vi "Overlay Circles.vi"(7 "Group":string, 8 "error in":errorcluster, 9 "Einstellungen":T1={"Farbe Kreis"=6618880, "Kreis ausfüllen?"=FALSE, "Bounding Rechteck anzeigen?"=FALSE, "Farbe Bounding Rechteck"=16711680}, 10 "Circles":T3(array[cluster]), 11 "Image in":T2) -> (0 "error out":errorcluster, 3 "Image out":T2)   [LabVIEW 2024]
uses:
  Kontaktmontagemodul.exe/1abvi3w/vi.lib/vision/Image Controls.llb/IMAQ Image.ctl
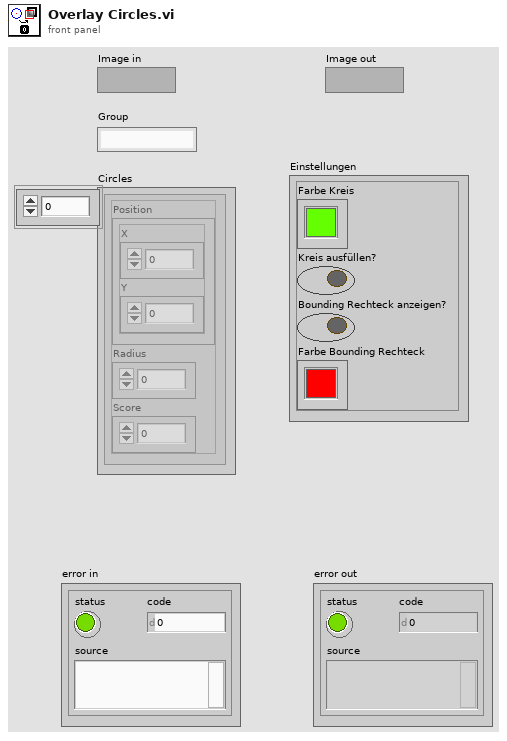
[diagram p1: front panel]
types:
  T1 = cluster{"Farbe Kreis":u32, "Kreis ausfüllen?":bool, "Bounding Rechteck anzeigen?":bool, "Farbe Bounding Rechteck":u32}
  T2 = typedef "IMAQ Image.ctl" = refnum<image>
  T3 = cluster{"Position":cluster{"X":sgl, "Y":sgl}, "Radius":dbl, "Score":dbl}[]
  T4 = cluster{"Left":i32, "Top":i32, "Right":i32, "Bottom":i32}
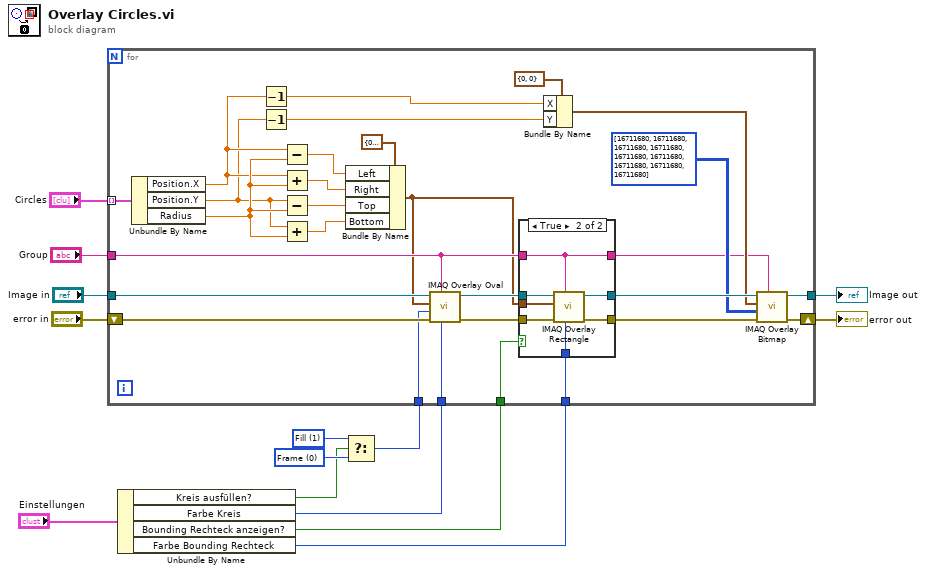
[diagram p0: block diagram]
diagram:
  w7 = u32 1 items=["Frame", "Fill"] ("Drawing Mode (Frame)")
  w8 = u32 0 items=["Frame", "Fill"] ("Drawing Mode (Frame)")
  n1 = Unbundle By Name("Einstellungen") -> ("Kreis ausfüllen?"=w5:bool, "Farbe Kreis"=w4:u32, "Bounding Rechteck anzeigen?"=w3:bool, "Farbe Bounding Rechteck"=w2:u32)
  n2 = Select(t=w7, s=w5, f=w8) -> (s? t:f=w6:u32)
  n3 = for {
    tunnel: "Circles" -> [w43] mode=indexing
    shift-right: [w15] -> w10
    shift-left: "error in" -> [w35]
    tunnel: "Image in" -> [w36]
    tunnel: [w17] -> w12
    tunnel: w4 -> [w23]
    tunnel: w6 -> [w22]
    tunnel: w3 -> [w21]
    tunnel: w2 -> [w20]
    tunnel: "Group" -> [w19]
    n4 = Unbundle By Name(w43) -> ("Position.X"=w28:sgl, "Position.Y"=w27:sgl, "Radius"=w41:dbl)
    n5 = Decrement(x=w28) -> (x-1=w26:sgl)
    n6 = Decrement(x=w27) -> (x-1=w25:sgl)
    n7 = Subtract(x=w28, y=w41) -> (x-y=w37:dbl)
    n8 = Add(x=w28, y=w41) -> (x+y=w38:dbl)
    n9 = Subtract(x=w27, y=w41) -> (x-y=w40:dbl)
    n10 = Add(x=w27, y=w41) -> (x+y=w39:dbl)
    n11 = Bundle By Name(cluster=T4 {"Left"=0, "Top"=0, "Right"=0, "Bottom"=0} ("Rectangle"), "Left"=w37, "Right"=w38, "Top"=w40, "Bottom"=w39) -> (w16:T4)
    n12 = call "IMAQ Overlay Oval"("Color"=w23, "Group"=w19, "error in (no error)"=w35, "Drawing Mode (Frame)"=w22, "Bounding Rectangle"=w16, "Image"=w36) -> ("error out"=w33:errorcluster, "Image Out"=w34:T2)  [unwired: 4 in]
    n13 = case shown="True" w21 {
      tunnel: w34 -> [w46 w53]
      tunnel: w33 -> [w45 w52]
      tunnel: w16 -> [_ w51]
      tunnel: [w46 w50] -> w32
      tunnel: [w45 w49] -> w31
      tunnel: w20 -> [_ w48]
      tunnel: w19 -> [w44 w47]
      tunnel: [w44 w47] -> w18
      frame False {
      }
      frame True {
        n14 = call "IMAQ Overlay Rectangle"("Color"=w48, "Group"=w47, "error in (no error)"=w52, "Rectangle"=w51, "Image"=w53) -> ("error out"=w49:errorcluster, "Image Out"=w50:T2)  [unwired: 5 in]
      }
    }
    n15 = Bundle By Name(cluster=cluster{"X":i32, "Y":i32} {"X"=0, "Y"=0} ("Top Left Point"), "X"=w26, "Y"=w25) -> (w24:cluster{"X":i32, "Y":i32})
    n16 = call "IMAQ Overlay Bitmap"("Group"=w18, "error in (no error)"=w31, "Bitmap"=u32[][] [[16711680, 16711680, 16711680], [16711680, 16711680, 16711680], [16711680, 16711680, 16711680]], "Top Left Point"=w24, "Image"=w32) -> ("error out"=w15:errorcluster, "Image Out"=w17:T2)  [unwired: 5 in]
  }
  "Image out" <- w12
  "error out" <- w10
